vi "Point getBounds.vi"(1 "points":T2[](array[typedef]) {"y" format="%.2f"; "x" format="%.2f"}, 5 "error in (no error)":errorcluster) -> (15 "boundsAdded":T1 {"height" format="%.2f"; "width" format="%.2f"; "y" format="%.2f"; "x" format="%.2f"}, 19 "error out":errorcluster)   [LabVIEW 2016]
doc: "contains"
uses:
  <resource>/Framework/Providers/Open_GDS/UML/General/Point/Point Point2D.ctl
  <resource>/Framework/Providers/Open_GDS/UML/General/Rectangle/Rectangle Rectangle2D.ctl
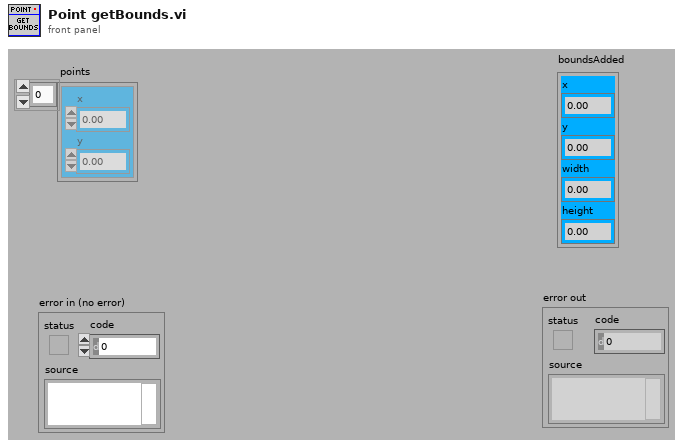
[diagram p1: front panel]
types:
  T1 = typedef "Rectangle Rectangle2D.ctl" = cluster{"x":dbl, "y":dbl, "width":dbl, "height":dbl}
  T2 = typedef "Point Point2D.ctl" = cluster{"x":dbl, "y":dbl}
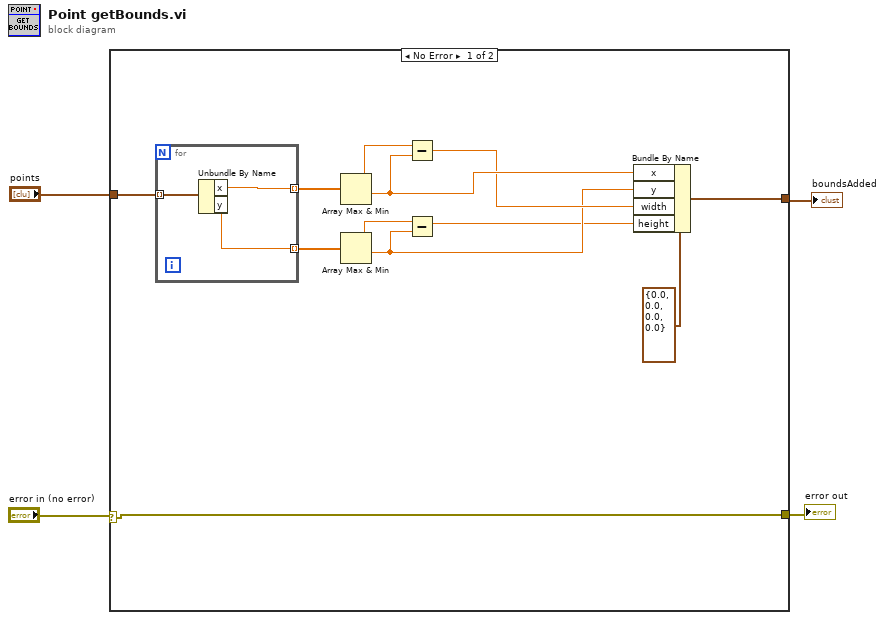
[diagram p0: block diagram]
diagram:
  n1 = case shown="No Error" "error in (no error)" {
    selector: "error in (no error)" -> [w16 w20]
    tunnel: [w16 w20] -> w4
    tunnel: "points" -> [w14 _]
    tunnel: [w15 _] -> w1
    frame No Error {
      n2 = for {
        tunnel: w14 -> [w19] mode=indexing
        tunnel: [w18] -> w13 mode=indexing
        tunnel: [w17] -> w7 mode=indexing
        n3 = Unbundle By Name(w19) -> ("x"=w18:dbl, "y"=w17:dbl)
      }
      n4 = Array Max & Min(array=w13) -> (max value=w11:dbl, min value=w10:dbl)  [unwired: 2 out]
      n5 = Array Max & Min(array=w7) -> (max value=w8:dbl, min value=w6:dbl)  [unwired: 2 out]
      n6 = Subtract(x=w11, y=w10) -> (x-y=w9:dbl)
      n7 = Subtract(x=w8, y=w6) -> (x-y=w5:dbl)
      n8 = Bundle By Name(cluster=T1 {"x"=0.0, "y"=0.0, "width"=0.0, "height"=0.0} ("boundsAdded"), "x"=w10, "y"=w6, "width"=w9, "height"=w5) -> (w15:T1)
    }
    frame Error {
    }
  }
  "error out" <- w4
  "boundsAdded" <- w1
